vi "test Abort Sub.vi"(11 "Test Case In":refnum<class "Tests Event MessengerM.lvclass">) -> (0 "error out":errorcluster, 3 "Test Case Out":refnum<class "Tests Event MessengerM.lvclass">)   [LabVIEW 2020, in "Tests Event MessengerM.lvclass"]
uses:
  Tests Event MessengerM.lvclass
  C:/Program Files/National Instruments/LabVIEW 2020/vi.lib/Astemes/LUnit/Test Case.lvclass
  <vilib>/Astemes/LUnit/Test Case.lvclass/Test Case.ctl
  <vilib>/Astemes/LUnit/Core/LUnit Test Case/Private/Append Fail Result.vi
  <vilib>/Astemes/LUnit/Core/LUnit Test Case/Private/Append Pass Result.vi
  <vilib>/Astemes/LUnit/Core/LUnit Test Case/Private/Run In UI.vi
  <vilib>/Utility/error.llb/Clear Errors.vi
  <extravilib>/ChannelInstances/Event MessengerM-c(str,var)/Instantiate.vi
  <extravilib>/ChannelInstances/Event MessengerM-c(str,var)/))Channel.vi
  <vilib>/Astemes/LUnit/Test Case.lvclass
  <extravilib>/ChannelInstances/Event MessengerM-c(str,var).lvlib
panel:
  out "cmd 2":string
  out "cmd":string
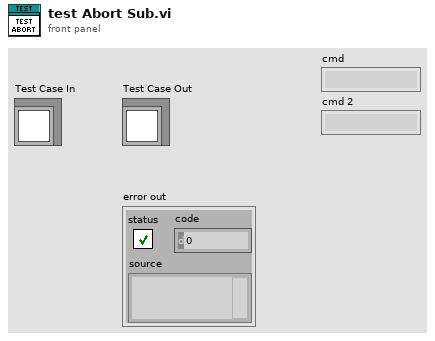
[diagram p1: front panel]
types:
  T1 = typedef "Event MessengerM-c(str,var).lvlib/))Channel.ctl" = refnum<queue>
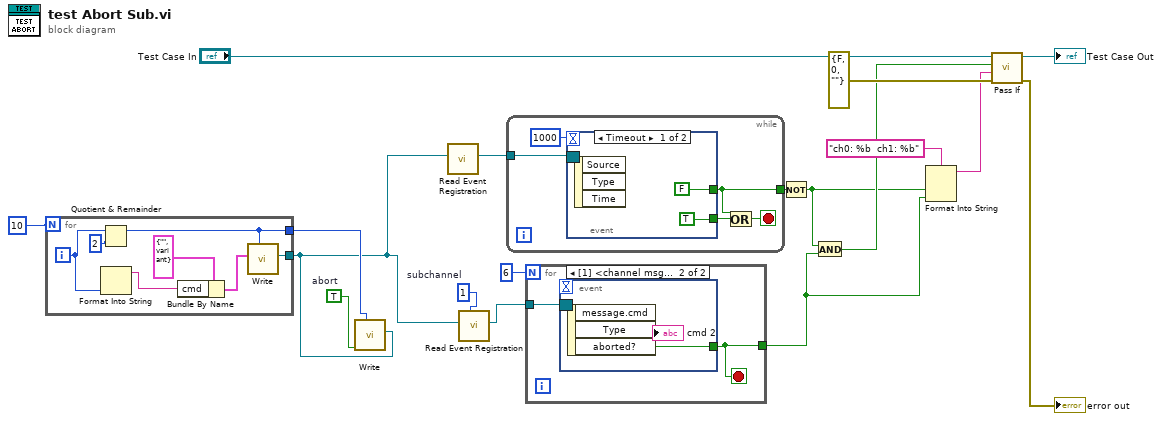
[diagram p0: block diagram]
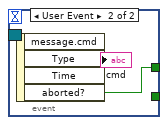
[diagram p2: hidden frame]
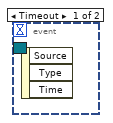
[diagram p3: hidden frame]
diagram:
  w5 = TRUE  # abort
  w1 = 1  # subchannel
  n1 = for {
    N: 10 -> [_]
    tunnel: [w20] -> w3
    tunnel: [w19] -> w6
    i -> [w23]
    n2 = Quotient & Remainder(x=w23, y=2) -> (x-y*floor(x/y)=w19:i32)  [unwired: 1 out]
    n3 = Format Into String(w23) -> (resulting string=w22:string)  [unwired: 3 in, 1 out]
    n4 = Bundle By Name(cluster=cluster{"cmd":string, "data":variant} {"cmd"="", "data"=variant} ("element"), "cmd"=w22) -> (w21:cluster{"cmd":string, "data":variant})
    n5 = call <extravilib>:"Write.vi"("subchannel (0)"=w19, "element"=w21) -> ("channel"=w20:T1)  [unwired: 8 in, 1 out]
  }
  n6 = call <extravilib>:"Write.vi"("channel"=w3, "subchannel (0)"=w6, "abort sub (F)"=w5) -> ()  [unwired: 8 in, 1 out]
  n7 = call <extravilib>:"Read Event Registration.vi"("channel"=w3) -> ("event registration refnum"=w4:refnum<event-registration>)  [unwired: 10 in]
  n8 = call <extravilib>:"Read Event Registration.vi"("subchannel (0)"=w1, "channel"=w3) -> ("event registration refnum"=w2:refnum<event-registration>)  [unwired: 9 in]
  n9 = while {
    tunnel: w4 -> [w30]
    tunnel: [w26] -> w13
    stop <- w27 stop-if-true
    n10 = event shown="[0] Timeout" {
      selector: w30 -> [_ _]
      dyn-events: _ -> [_ _]
      timeout: 1000 -> [_ _]
      tunnel: [FALSE ("aborted?") w33] -> w26
      tunnel: [TRUE _] -> w28
      event Timeout {
        n11 = event-data() -> ()  [unwired: 1 in, 3 out]
      }
      event User Event {
        n12 = event-data() -> ("message.cmd"=→"cmd":string, "aborted?"=w33:bool)  [unwired: 1 in, 2 out]
      }
    }
    n13 = Or(x=w26, y=w28) -> (x .or. y?=w27:bool)
  }
  n14 = for {
    N: 6 -> [_]
    tunnel: w2 -> [w36]
    tunnel: [w35] -> w8
    stop <- w35 stop-if-true
    n15 = event shown="[1] <channel msg>: User Event" {
      selector: w36 -> [_ _]
      dyn-events: _ -> [_ _]
      timeout: _ -> [_ _]
      tunnel: [_ w37] -> w35
      event Timeout {
        n16 = event-data() -> ()  [unwired: 1 in, 3 out]
      }
      event User Event {
        n17 = event-data() -> ("message.cmd"=→"cmd 2":string, "aborted?"=w37:bool)  [unwired: 1 in, 1 out]
      }
    }
  }
  n18 = Not(x=w13) -> (.not. x?=w7:bool)
  n19 = And(x=w7, y=w8) -> (x .and. y?=w11:bool)
  n20 = Format Into String(format string="ch0: %b  ch1: %b", w7, w8) -> (resulting string=w9:string)  [unwired: 2 in, 1 out]
  n21 = call <vilib>:"Pass If.vi"("error in (no error)"=errorcluster {"status"=FALSE, "code"=0, "source"=""}, "Message"=w9, "Pass?"=w11, "LUnit Test Case In"="Test Case In") -> ("error out"=→"error out":errorcluster, "LUnit Test Case Out"=→"Test Case Out":refnum<class "Tests Event MessengerM.lvclass">)  [unwired: 6 in]
